vi "Check if Anlytics Enabled.vi"(8 "error in":errorcluster, 11 "Default JSON \nVariant in":variant) -> (0 "error out":errorcluster, 3 "Analytics Enabled?":bool)   [LabVIEW 2015, in "ZenGage v3.0 UI.lvclass"]
uses:
  ZenGage v3.0 UI.lvclass
panel:
  out "Error Message":string
  out "VClusterOut":variant
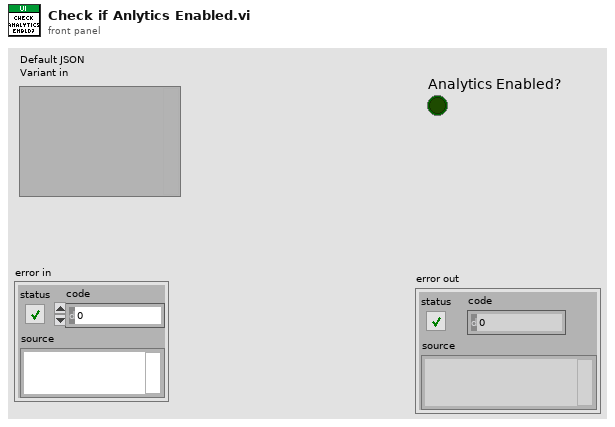
[diagram p1: front panel]
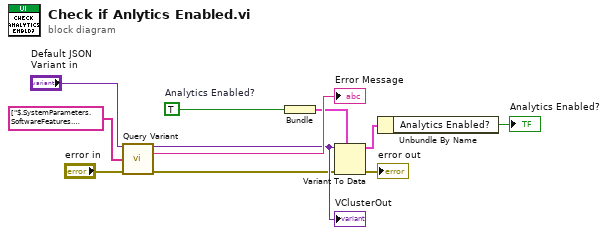
[diagram p0: block diagram]
diagram:
  w7 = TRUE  # Analytics Enabled?
  n1 = call <vilib>:"Query Variant.vi"("VCluster in"="Default JSON \nVariant in", "pathList"=string[] ["$.SystemParameters.SoftwareFeatures.AnalyticsEnable"], "error IO"="error in") -> ("VCluster\n out"=w8:variant, "Error Message"=→"Error Message":string, "error out"=w1:errorcluster)  [unwired: 9 in, 1 out]
  "VClusterOut" <- w8
  n2 = Bundle("Analytics Enabled?"=w7) -> (w6:cluster{"Analytics Enabled?":bool})  [unwired: 1 in]
  n3 = Variant To Data(error in=w1, type=w6, Variant=w8) -> (data=w5:cluster{"Analytics Enabled?":bool}, error out=→"error out":errorcluster)
  n4 = Unbundle By Name(w5) -> ("Analytics Enabled?"=→"Analytics Enabled?":bool)
